vi "command_codes.vi"(1 "command code enum":T1) -> (0 "command code":string)   [LabVIEW 2021]
uses:
  typedefs/command.ctl
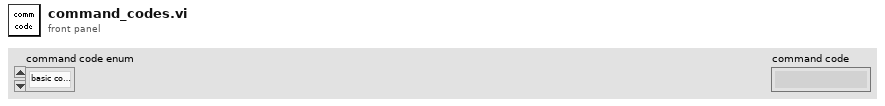
[diagram p1: front panel]
types:
  T1 = typedef "command.ctl" = enum16{"basic configuration", "test configuration", "converter configuration", "reset", "start", "next cell", "next state"}
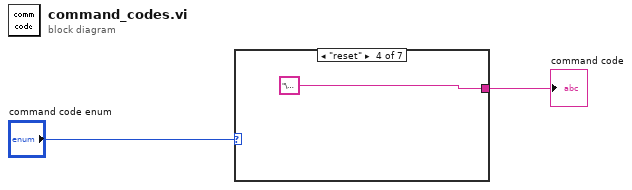
[diagram p0: block diagram]
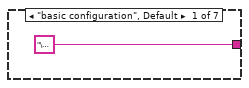
[diagram p2: hidden frame]
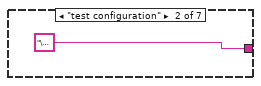
[diagram p3: hidden frame]
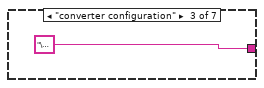
[diagram p4: hidden frame]
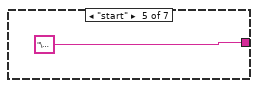
[diagram p5: hidden frame]
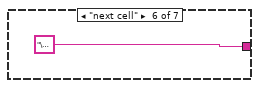
[diagram p6: hidden frame]
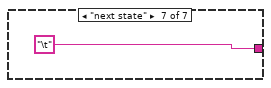
[diagram p7: hidden frame]
diagram:
  n1 = case shown="\"reset\"" "command code enum" {
    tunnel: ["\u0003" "\u0005" "\u0007" "\u0003" "\u0005" "\u0007" "\t"] -> w2
    frame "basic configuration", Default {
    }
    frame "test configuration" {
    }
    frame "converter configuration" {
    }
    frame "reset" {
    }
    frame "start" {
    }
    frame "next cell" {
    }
    frame "next state" {
    }
  }
  "command code" <- w2
